vi "Get Parameter.vi"(8 "error in (no error)":errorcluster, 11 "Simulated ParameterDevice in":refnum<class "Simulated ParameterDevice.lvclass">) -> (0 "error out":errorcluster, 2 "Parameter out":refnum<class "AbstractData.lvclass">, 3 "Simulated ParameterDevice out":refnum<class "Simulated ParameterDevice.lvclass">)   [LabVIEW 2014, in "Simulated ParameterDevice.lvclass"]
uses:
  Simulated ParameterDevice.lvclass
  Framework/Model/Data/AbstractData/AbstractData.lvclass
  Framework/Model/Data/DataSingleElement/DataSingleElement.lvclass
  Simulated ParameterDevice.lvclass/Simulated ParameterDevice.ctl
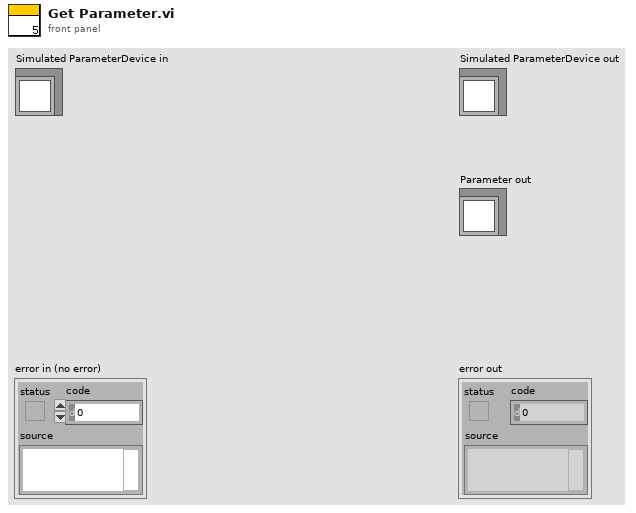
[diagram p1: front panel]
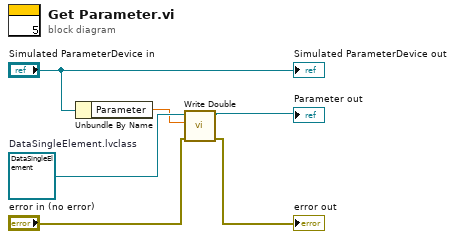
[diagram p0: block diagram]
diagram:
  w4 = refnum<class "DataSingleElement.lvclass"> refnum  # DataSingleElement.lvclass
  n1 = Unbundle By Name("Simulated ParameterDevice in") -> ("Parameter"=w3:dbl)
  n2 = call "Write Double.vi"("error in (no error)"="error in (no error)", "value"=w3, "DataSingleElement in"=w4) -> ("error out"=→"error out":errorcluster, "DataSingleElement out"=→"Parameter out":refnum<class "DataSingleElement.lvclass">)  [unwired: 7 in]
  "Simulated ParameterDevice out" <- "Simulated ParameterDevice in"
